vi "GEA2 Serial Get Destination Address.vi"(8 "Error In":errorcluster, 9 "Source Destination":T1 {"Destination" format="%x"; "Source" format="%x"}, 10 "Current Read Index":i32, 11 "ReadArray":u8[](array[numeric])) -> (0 "Error Out":errorcluster, 1 "Destination Read":u8 format="%.0x", 2 "CRC Array":u8[](array[numeric]), 3 "Current Read Index":i32, 4 "Message":bool)   [LabVIEW 2014]
uses:
  Type Definitions/Source Destination Control.ctl
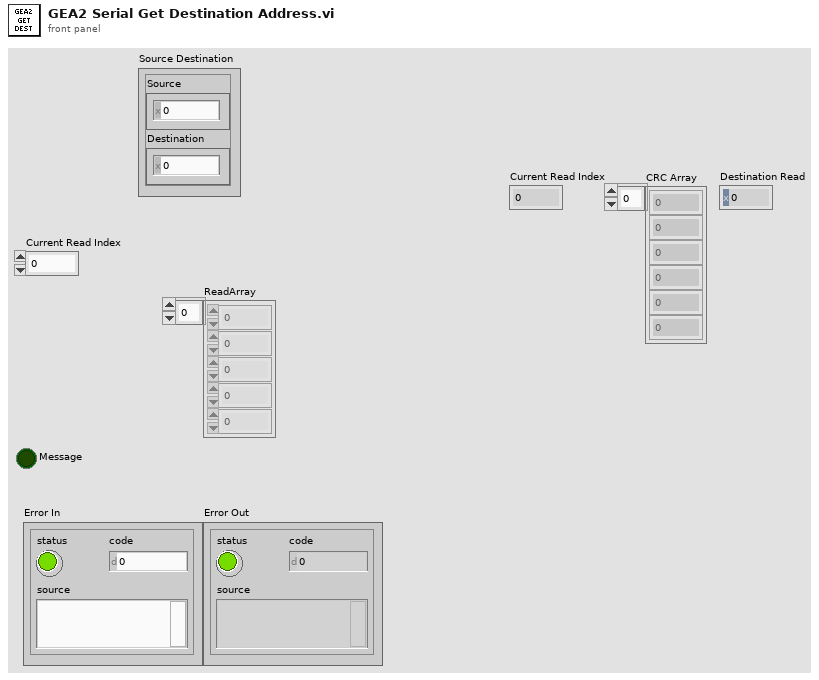
[diagram p1: front panel]
types:
  T1 = typedef "Source Destination Control.ctl" = cluster{"Source":u8, "Destination":u8}
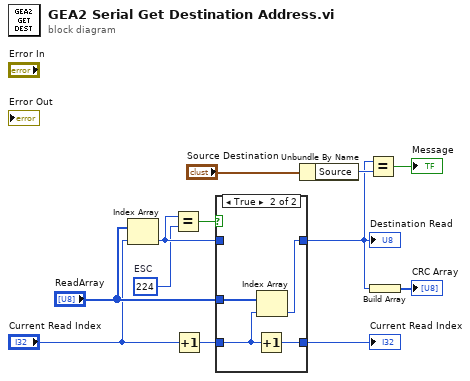
[diagram p0: block diagram]
diagram:
  w3 = u8 224  # ESC
  n1 = Index Array(array="ReadArray", index="Current Read Index") -> (element=w10:u8)
  n2 = Equal?(x=w10, y=w3) -> (x = y?=w4:bool)
  n3 = Increment(x="Current Read Index") -> (x+1=w7:i32)
  n4 = case shown="True" w4 {
    tunnel: [w14 w15] -> w8
    tunnel: [w13 w17] -> w5
    tunnel: "ReadArray" -> [_ w18]
    tunnel: w7 -> [w13 w16]
    tunnel: w10 -> [w14 _]
    frame False {
    }
    frame True {
      n5 = Increment(x=w16) -> (x+1=w17:i32)
      n6 = Index Array(array=w18, index=w16) -> (element=w15:u8)
    }
  }
  "Destination Read" <- w8
  "Current Read Index" <- w5
  n7 = Unbundle By Name("Source Destination") -> ("Source"=w12:u8)
  n8 = Equal?(x=w8, y=w12) -> (x = y?=→"Message":bool)
  n9 = Build Array(w8) -> (→"CRC Array":u8[])
